vi "New.vi"(8 "error in (no error)":errorcluster, 11 "Picture Ref":refnum<vi>) -> (0 "error out":errorcluster, 3 "BetterTreeBar out":refnum<class "BetterHorizontalBar.lvclass">)   [LabVIEW 2020, in "BetterDragAndDrop.lvlib" / "BetterHorizontalBar.lvclass"]
uses:
  BetterHorizontalBar.lvclass
  SubVIs/Horizontal Bar Enumeration.ctl
  BetterHorizontalBar.lvclass/BetterHorizontalBar.ctl
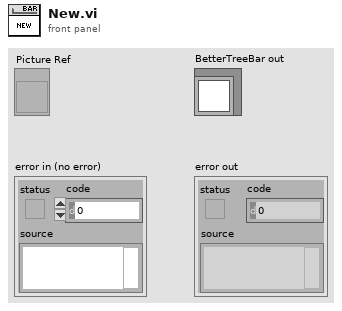
[diagram p1: front panel]
types:
  T1 = typedef "BetterDragAndDrop.lvlib/BetterHorizontalBar.lvclass/Horizontal Bar Enumeration.ctl" = enum16{"None", "only bar", "tilda up"}
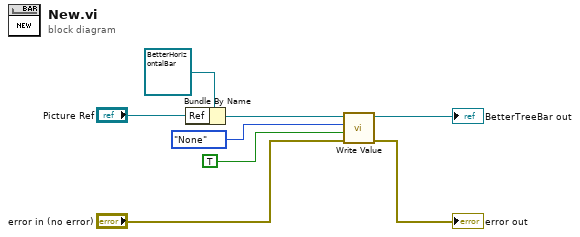
[diagram p0: block diagram]
diagram:
  n1 = Bundle By Name(cluster=refnum<class "BetterHorizontalBar.lvclass"> refnum ("BetterTreeBar out"), "Ref"="Picture Ref") -> (w6:refnum<class "BetterHorizontalBar.lvclass">)
  n2 = call "Write Value.vi"("error in (no error)"="error in (no error)", "Force draw? (F)"=TRUE, "New Value"=Horizontal_Bar_Enumeration."None", "BetterTreeBar in"=w6) -> ("error out"=→"error out":errorcluster, "BetterTreeBar out"=→"BetterTreeBar out":refnum<class "BetterHorizontalBar.lvclass">)  [unwired: 6 in]
